vi "Do.vi"(8 "error in (no error)":errorcluster, 10 "Actor in":refnum<class "Actor.lvclass">, 11 "Launch UI Message":refnum<class "Launch User Interface Msg.lvclass">) -> (0 "error out":errorcluster, 2 "Actor out":refnum<class "Actor.lvclass">)   [LabVIEW 2016, in "Controller Actor.lvlib" / "Launch User Interface Msg.lvclass"]
uses:
  <userlib>/Common Components/Controller/Messages/Launch UI Message/Launch User Interface Msg.lvclass
  <vilib>/ActorFramework/Actor/Actor.lvclass
  <userlib>/Common Components/Controller/Controller.lvclass
  C:/Program Files (x86)/National Instruments/LabVIEW 2016/vi.lib/ActorFramework/Actor/Actor.lvclass
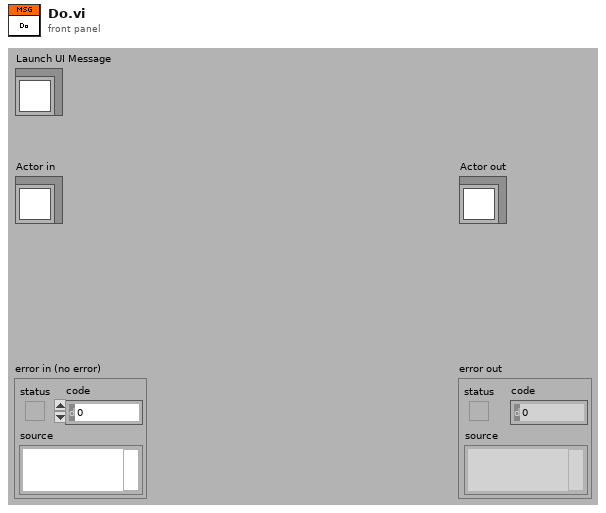
[diagram p1: front panel]
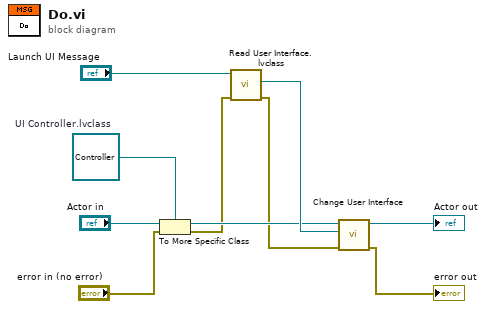
[diagram p0: block diagram]
diagram:
  w10 = refnum<class "Controller.lvclass"> refnum  # UI Controller.lvclass
  n1 = To More Specific Class(target class=w10, reference="Actor in", error in="error in (no error)") -> (specific class reference=w6:refnum<class "Controller.lvclass">, error out=w3:errorcluster)
  n2 = call <userlib>:"Read User Interface.lvclass.vi"("error in (no error)"=w3, "Launch UI Message in"="Launch UI Message") -> ("error out"=w2:errorcluster, "User Interface.lvclass"=w7:refnum<class "UI.lvclass">)  [unwired: 7 in, 1 out]
  n3 = call <userlib>:"Change User Interface.vi"("error in (no error)"=w2, "User Interface.lvclass"=w7, "Test Step Controller in"=w6) -> ("error out"=→"error out":errorcluster, "Test Step Controller out"=→"Actor out":refnum<class "Controller.lvclass">)  [unwired: 7 in]
